vi "Close.vi"(8 "error in":errorcluster, 11 "AI Current DAQmx Cont CFG in":refnum<class "AI Current DAQmx Cont CFG.lvclass">) -> (0 "error out":errorcluster, 3 "AI Current DAQmx Cont CFG out":refnum<class "AI Current DAQmx Cont CFG.lvclass">)   [LabVIEW 2024, in "AI Current DAQmx Cont CFG.lvclass"]
uses:
  AI Current DAQmx Cont CFG.lvclass
  AI Current DAQmx Cont CFG.lvclass/AI Current DAQmx Cont CFG.ctl
  DAQmx Base CFG/DAQmx Base CFG.lvclass
  Buffers/BufferLossless/BufferLossless.lvclass
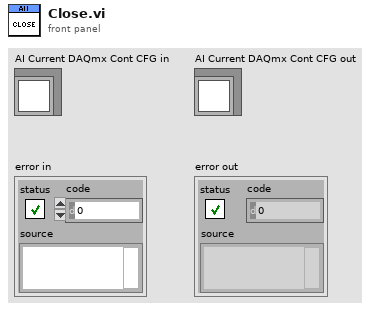
[diagram p1: front panel]
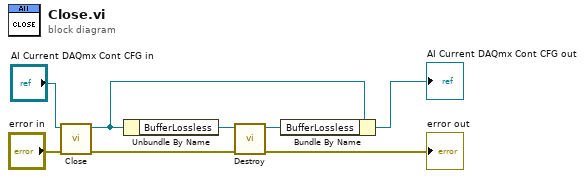
[diagram p0: block diagram]
diagram:
  n1 = call-parent "Close.vi"("error in"="error in", "DAQmx Base CFG in"="AI Current DAQmx Cont CFG in") -> ("error out"=w5:errorcluster, "DAQmx Base CFG out"=w3:refnum<class "AI Current DAQmx Cont CFG.lvclass">)  [unwired: 8 in]
  n2 = Unbundle By Name(w3) -> ("BufferLossless"=w6:refnum<class "BufferLossless.lvclass">)
  n3 = call "Destroy.vi"("error in"=w5, "BufferLossless in"=w6) -> ("error out"=→"error out":errorcluster, "BufferLossless out"=w4:refnum<class "BufferLossless.lvclass">)  [unwired: 8 in]
  n4 = Bundle By Name(cluster=w3, "BufferLossless"=w4) -> (→"AI Current DAQmx Cont CFG out":refnum<class "AI Current DAQmx Cont CFG.lvclass">)
